vi "Read Address.vi"(7 "Number of Addresses to read (1)":u8=1, 8 "error in (no error)":errorcluster, 9 "Address number (0)":u8 max=49, 10 "Motor ID (0)":u8, 11 "Dynamixel Motor in":refnum<class "Dynamixel Motor.lvclass">) -> (0 "error out":errorcluster, 1 "Motor Error Status":T1, 2 "Data Read":u8[](array[numeric]), 3 "Dynamixel Motor out":refnum<class "Dynamixel Motor.lvclass">)   [LabVIEW 2016, in "Dynamixel Motor.lvclass"]
doc: "Reads an arbitrary number of consecutive addresses from a motor's register. This is a Low-Level VI that is used by other VIs."
uses:
  <instrlib>/Dynamixel Motor/HAIOL/Dynamixel Motor.lvclass
  <instrlib>/Dynamixel Motor/Public/Motor Operation/Low Level/Alarm Setting.ctl
  <instrlib>/Dynamixel Motor/Dynamixel Motor.lvlib
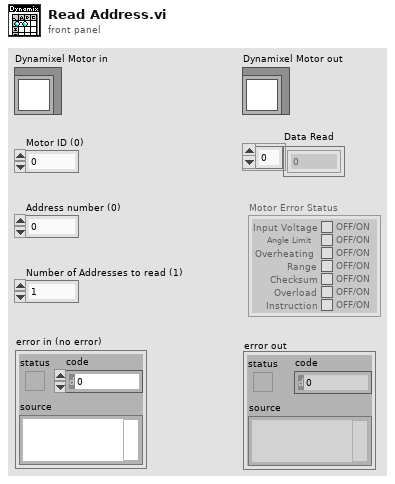
[diagram p1: front panel]
types:
  T1 = typedef "Dynamixel Motor.lvlib/Alarm Setting.ctl" = cluster{"Input Voltage":bool, "Angle Limit":bool, "Overheating ":bool, "Range":bool, "Checksum":bool, "Overload":bool, "Instruction":bool}
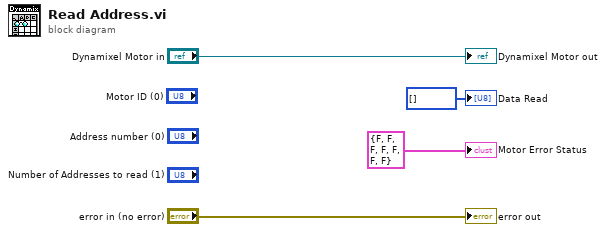
[diagram p0: block diagram]
diagram:
  "error out" <- "error in (no error)"
  "Dynamixel Motor out" <- "Dynamixel Motor in"
  "Motor Error Status" <- T1 {"Input Voltage"=FALSE, "Angle Limit"=FALSE, "Overheating "=FALSE, "Range"=FALSE, "Checksum"=FALSE, "Overload"=FALSE, "Instruction"=FALSE} ("Motor Error Status")
  "Data Read" <- u8[] [] ("Data Read")
